vi "templates ordered list.vi"(6 "sxUsername":string, 8 "error in (no error)":errorcluster, 10 "sxTemplateId (\"\")":string, 11 "Connection Refnum":T1) -> (0 "error out":errorcluster, 2 "Templates List":string, 3 "Connection Refnum":T1)   [LabVIEW 2011]
uses:
  SI.LIB/ODBC/SQL Controls/Connection Refnum.ctl
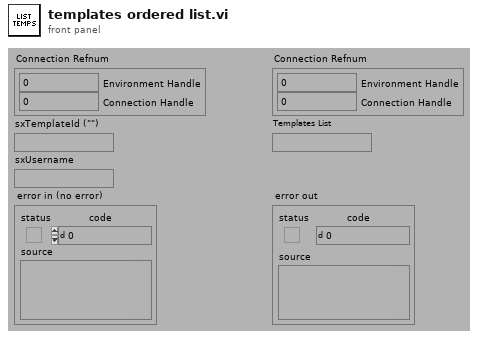
[diagram p1: front panel]
types:
  T1 = typedef "Connection Refnum.ctl" = cluster{"Environment Handle":i32, "Connection Handle":i32}
  T2 = typedef "Template Record.ctl" = cluster{"ixTemplate":i32, "sxTemplateId":string, "sDescription":string, "sCreator":string, "tCreationDate":timestamp, "sModifier":string, "tModifiedDate":timestamp, "sType":string, "sStyle":string, "sFormat":string, "dWidth":dbl, "dHeight":dbl, "sFilename":string, "sScript":string, "sLayout":string, "sEditor":string, "sStyleProcess":string}
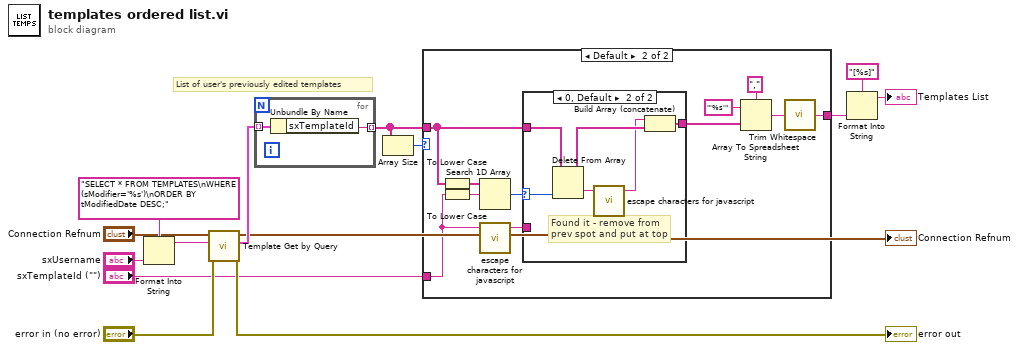
[diagram p0: block diagram]
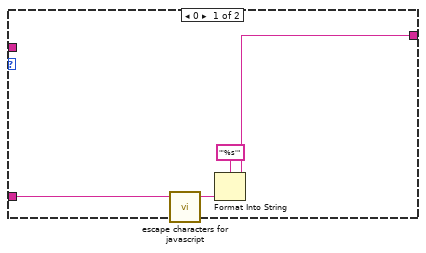
[diagram p2: hidden frame]
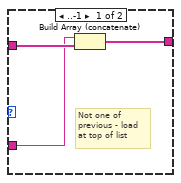
[diagram p3: hidden frame]
diagram:
  # "List of user's previously edited templates"
  n1 = Format Into String(format string="SELECT * FROM TEMPLATES\nWHERE (sModifier='%s')\nORDER BY tModifiedDate DESC;", "sxUsername") -> (resulting string=w13:string)  [unwired: 2 in, 1 out]
  n2 = call "Template Get by Query.vi"("error in (no error)"="error in (no error)", "Template Query (\"\")"=w13, "Connection Refnum"="Connection Refnum") -> ("error out"=→"error out":errorcluster, "Records"=w12:T2[], "Connection Refnum"=→"Connection Refnum":T1)  [unwired: 6 out]
  n3 = for {
    tunnel: w12 -> [w16] mode=indexing
    tunnel: [w15] -> w3 mode=indexing
    n4 = Unbundle By Name(w16) -> ("sxTemplateId"=w15:string)
  }
  n5 = Array Size(array=w3) -> (size(s)=w1:i32)
  n6 = case shown="Default" w1 {
    tunnel: "sxTemplateId (\"\")" -> [w18 w25]
    tunnel: [w17 w22] -> w4
    tunnel: w3 -> [_ w21]
    frame 0 {
      n7 = call "escape characters for javascript.vi"("String (\"\")"=w18) -> ("escaped String"=w20:string)  [unwired: 4 out]
      n8 = Format Into String(format string="'%s'", w20) -> (resulting string=w17:string)  [unwired: 2 in, 1 out]
    }
    frame Default {
      n9 = To Lower Case(string=w21) -> (all lower case string=w26:string[])
      n10 = To Lower Case(string=w25) -> (all lower case string=w28:string)
      n11 = Search 1D Array(1D array=w26, element=w28) -> (index of element=w27:i32)  [unwired: 1 out]
      n12 = call "escape characters for javascript.vi"("String (\"\")"=w25) -> ("escaped String"=w24:string)  [unwired: 4 out]
      n13 = case shown="0, Default" w27 {
        selector: w27 -> [_ w39]
        tunnel: w21 -> [w34 w40]
        tunnel: w24 -> [w33 _]
        tunnel: [w32 w37] -> w23
        frame ..-1 {
          # "Not one of \nprevious - load\nat top of list"
          n14 = Build Array (concatenate)(w33, w34) -> (w32:string[])
        }
        frame 0, Default {
          # "Found it - remove from\nprev spot and put at top"
          n15 = Delete From Array(array=w40, index=w39) -> (deleted portion=w36:string, array with subset deleted=w38:string[])  [unwired: 1 in]
          n16 = call "escape characters for javascript.vi"("String (\"\")"=w36) -> ("escaped String"=w35:string)  [unwired: 4 out]
          n17 = Build Array (concatenate)(w35, w38) -> (w37:string[])
        }
      }
      n18 = Array To Spreadsheet String(delimiter (Tab)=",", array=w23, 3:"'%s'") -> (spreadsheet string=w29:string)
      n19 = call <vilib>:"Trim Whitespace.vi"("string"=w29) -> ("trimmed string"=w22:string)  [unwired: 1 in]
    }
  }
  n20 = Format Into String(format string="[%s]", w4) -> (resulting string=→"Templates List":string)  [unwired: 2 in, 1 out]
